vi "BoolTrueFalseGen.vi"(7 "Error in":errorcluster, 9 "Énum":enum16{"TrueFalse", "YesNo", "OnOff"}(ring), 10 "Bool":bool) -> (0 "Error out":errorcluster, 3 "TrueFalse":string="Init")   [LabVIEW 2019]
doc: "Ce VI ouvre le fichier de sauvegarde des modèles et lit les positions du modèle spécifié."
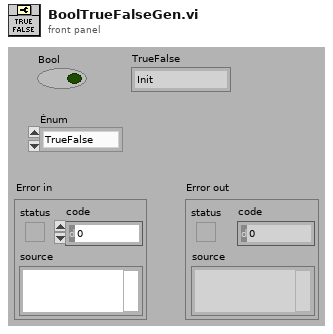
[diagram p1: front panel]
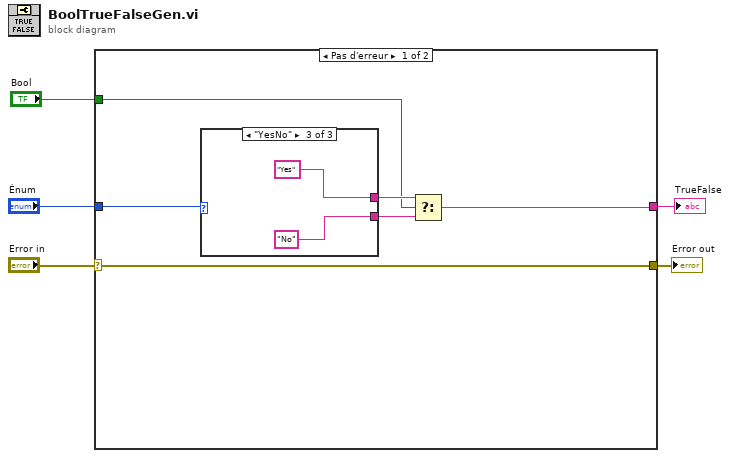
[diagram p0: block diagram]
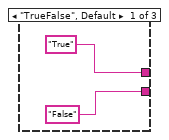
[diagram p2: hidden frame]
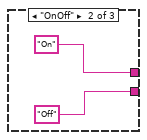
[diagram p3: hidden frame]
diagram:
  n1 = case shown="Pas d'erreur" "Error in" {
    selector: "Error in" -> [w11 w18]
    tunnel: [w11 w18] -> w5
    tunnel: "Bool" -> [w8 _]
    tunnel: "Énum" -> [w7 _]
    tunnel: [w6 _] -> w1
    frame No Error {
      n2 = case shown="\"YesNo\"" w7 {
        tunnel: ["True" "On" "Yes"] -> w10
        tunnel: ["False" "Off" "No"] -> w9
        frame "TrueFalse", Default {
        }
        frame "OnOff" {
        }
        frame "YesNo" {
        }
      }
      n3 = Select(t=w10, s=w8, f=w9) -> (s? t:f=w6:string)
    }
    frame Error {
    }
  }
  "Error out" <- w5
  "TrueFalse" <- w1
